vi "State Machine.vi"() -> ()   [LabVIEW 2015]
uses:
  Warning.ctl
  <vilib>/ErrorRing/Error Ring.xnode
panel:
  out "value voltage":dbl caption="Current Value (V)" format="%#.2g"
  out "Meter":dbl(knob) caption="Voltage" scale=0.0..12.0
  out "Low Link Quality Voltage":bool caption="Low"
  out "timed out?\nSignal potentiometer":bool caption="Timeout"
  out "Low Battery Voltage":bool caption="Low"
  out "timed out?\nBattery potentiometer":bool caption="Timeout"
  out "Signal > 75 %":bool
  out "Signal > 50 %":bool
  out "Signal > 25%":bool
  out "Signal > 0%":bool
  out "Battery > 75 %":bool
  out "Battery > 50 %":bool
  out "Battery > 25%":bool
  out "Battery > 0%":bool
  in  "upper and lower voltage threshold":cluster{dbl, dbl}(knob)={0.0, 12.0} caption="Voltage Threshold" scale=0.0..12.0
  out "Too High Voltage":bool
  out "Too Low Voltage":bool
  out "Low Link Quality Temp":bool caption="Low"
  out "timed out?\nLink Quality\nThermometer":bool caption="Timeout"
  out "Low Battery Temp":bool caption="Low"
  out "timed out?\nBattery Thermometer":bool caption="Timeout"
  out "Date":timestamp format="%<%d/%m/%y>T"
  out "Time":timestamp format="%<%H:%M>T"
  in  "Start/ pause":bool
  in  "Stop button":bool
  in  "upper and lower temp threshold":cluster{dbl, dbl}(knob)={0.0, 30.0} caption="Temperature Threshold" scale=-20.0..60.0
  out "Thermometer":dbl(slide) caption="Temperature" scale=-20.0..60.0
  in  "Error In":errorcluster
  out "Too hot":bool
  out "Too cold":bool
  out "min volt":sgl caption="Minimum (V)" format="%#.2g"
  out "max volt":sgl caption="Maximum (V)" format="%#.2g"
  out "mean volt":T1 caption="Mean (V)" format="%#.2g"
  out "voltage":sgl(graph)
  out "min temp":sgl caption="Minimum (°C)" format="%#.2g"
  out "max temp":sgl caption="Maximum (°C)" format="%#.2g"
  out "mean temp":sgl caption="Mean (°C)" format="%#.2g"
  out "temperature":sgl(graph)
  out "Signal > 75 % Temp":bool
  out "Signal > 50 % Temp":bool
  out "Signal > 25% Temp":bool
  out "Signal > 0% Temp":bool
  out "Battery > 75 % Temp":bool
  out "Battery > 50 % Temp":bool
  out "Battery > 25% Temp":bool
  out "Battery > 0% Temp":bool
  out "Low radio signal\nfor potentiometer":errorcluster
  out "Low Battery\nfor potentiometer":errorcluster
  out "No Signal \non thermometer":errorcluster
  out "No Signal\non potentiometer":errorcluster
  out "Low radio signal\nfor thermometer":errorcluster
  out "Low Battery\nfor thermometer":errorcluster
  # "Thermometer"
  # "Potentiometer"
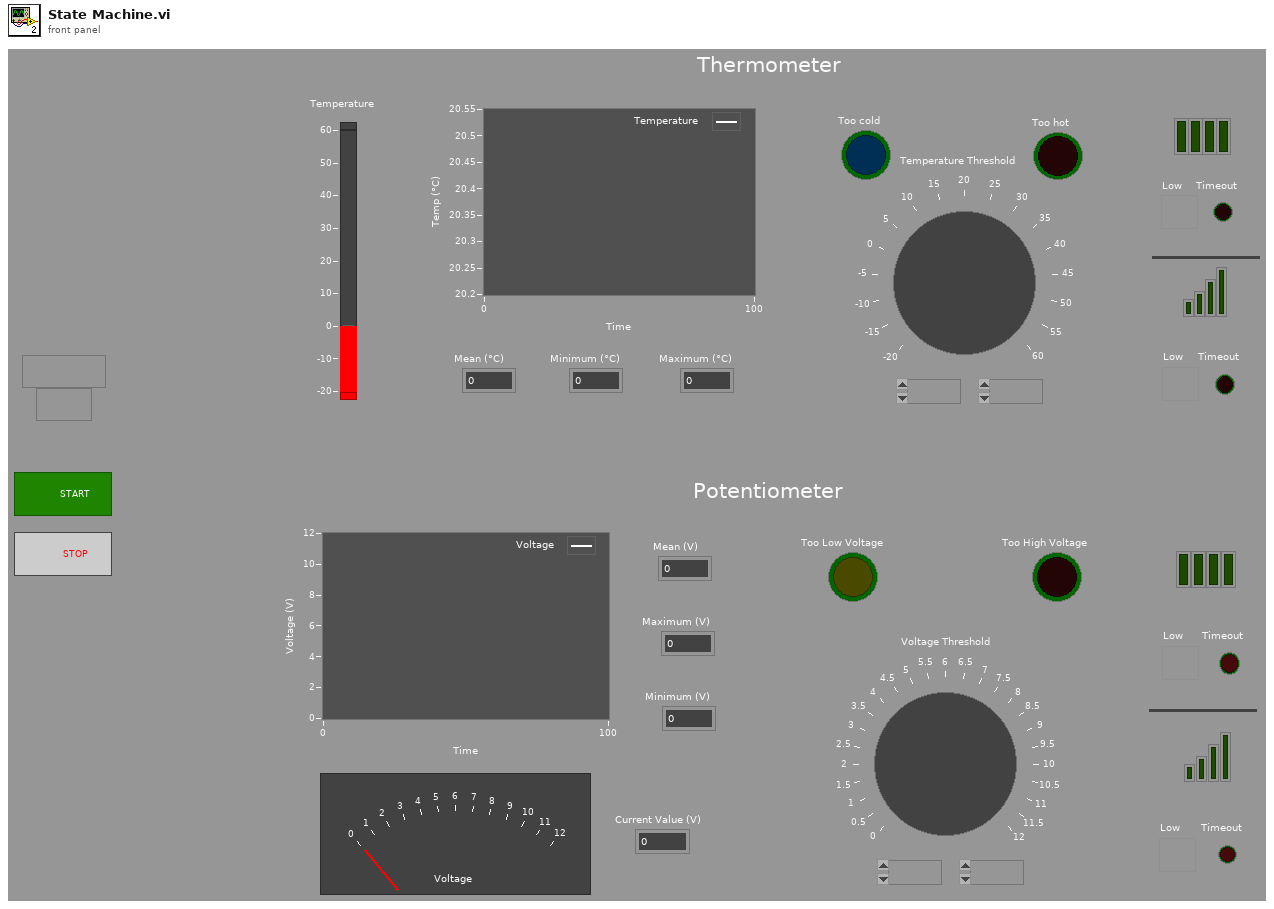
[diagram p1: front panel]
types:
  T1 = typedef "Warning.ctl" = sgl
  T2 = enum16{"open", "replace", "create", "open or create", "replace or create", "replace or create with confirmation"}
  T3 = enum8{"Enabled", "Disabled", "Disabled and Grayed Out"}
  T4 = enum16{"Error and Alert handler", "Acquisition, calculations and save"}
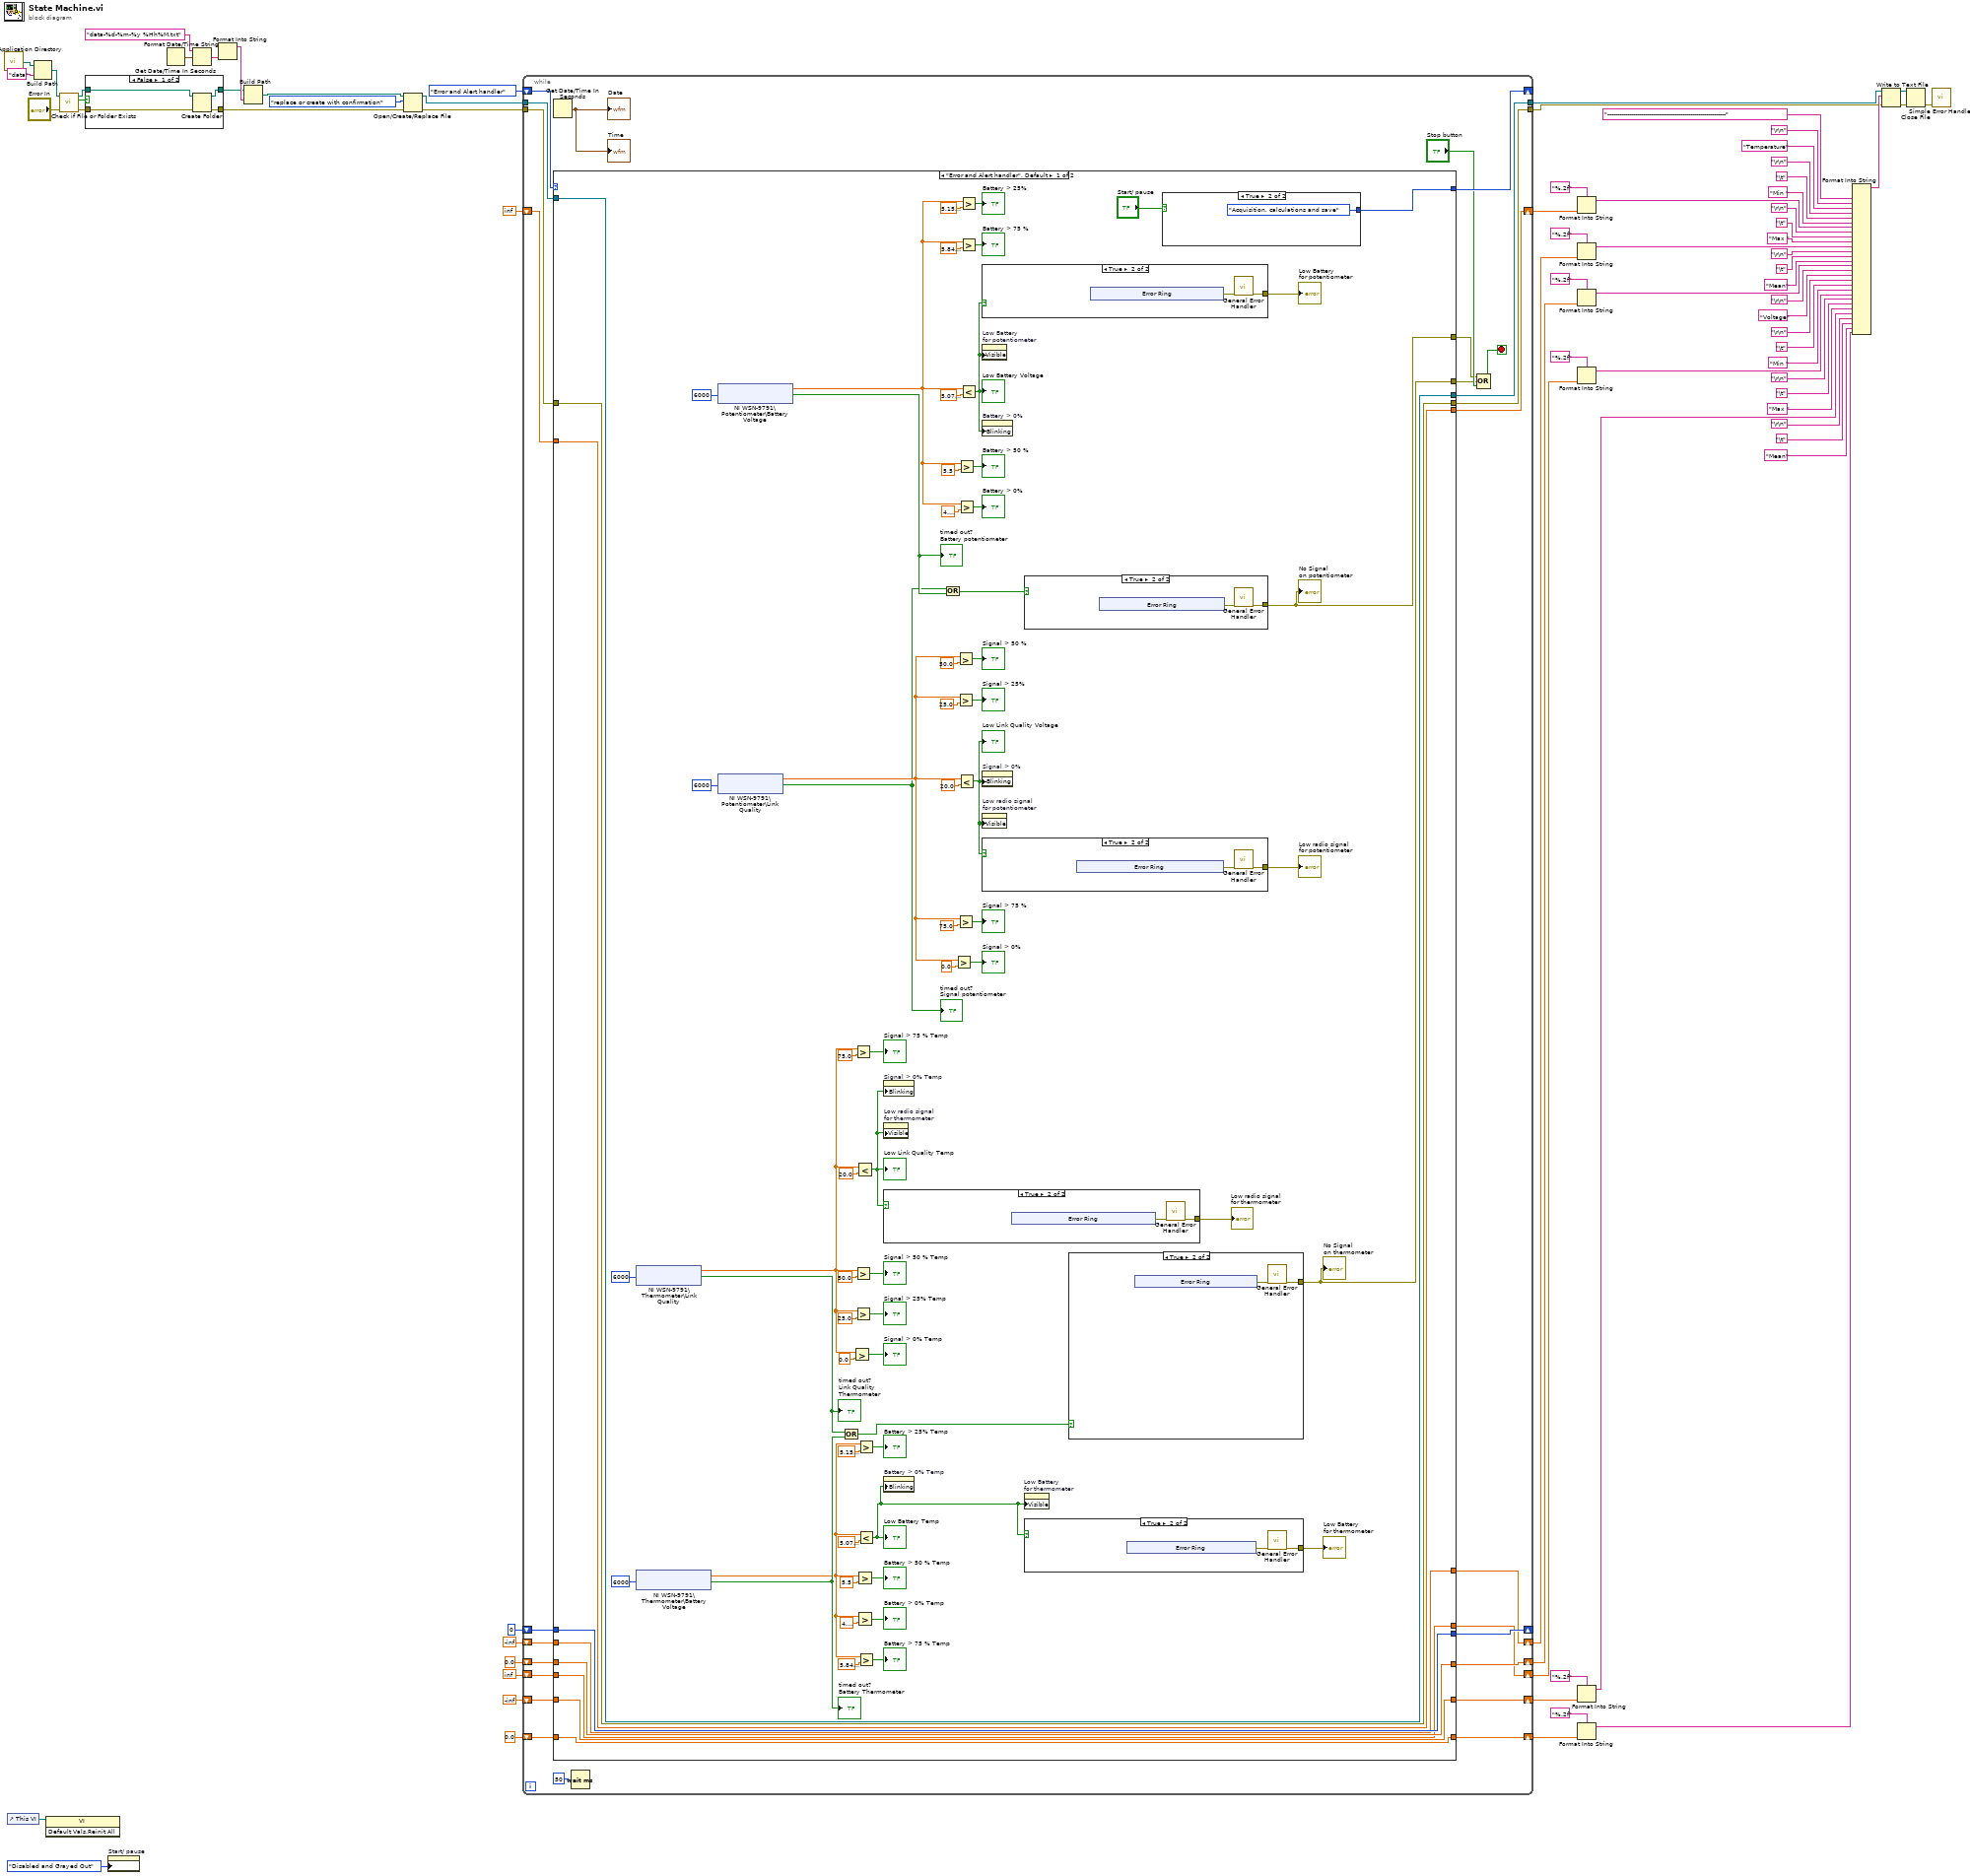
[diagram p0: block diagram]
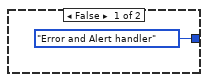
[diagram p3: hidden frame]
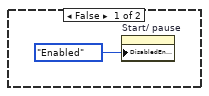
[diagram p7: hidden frame]
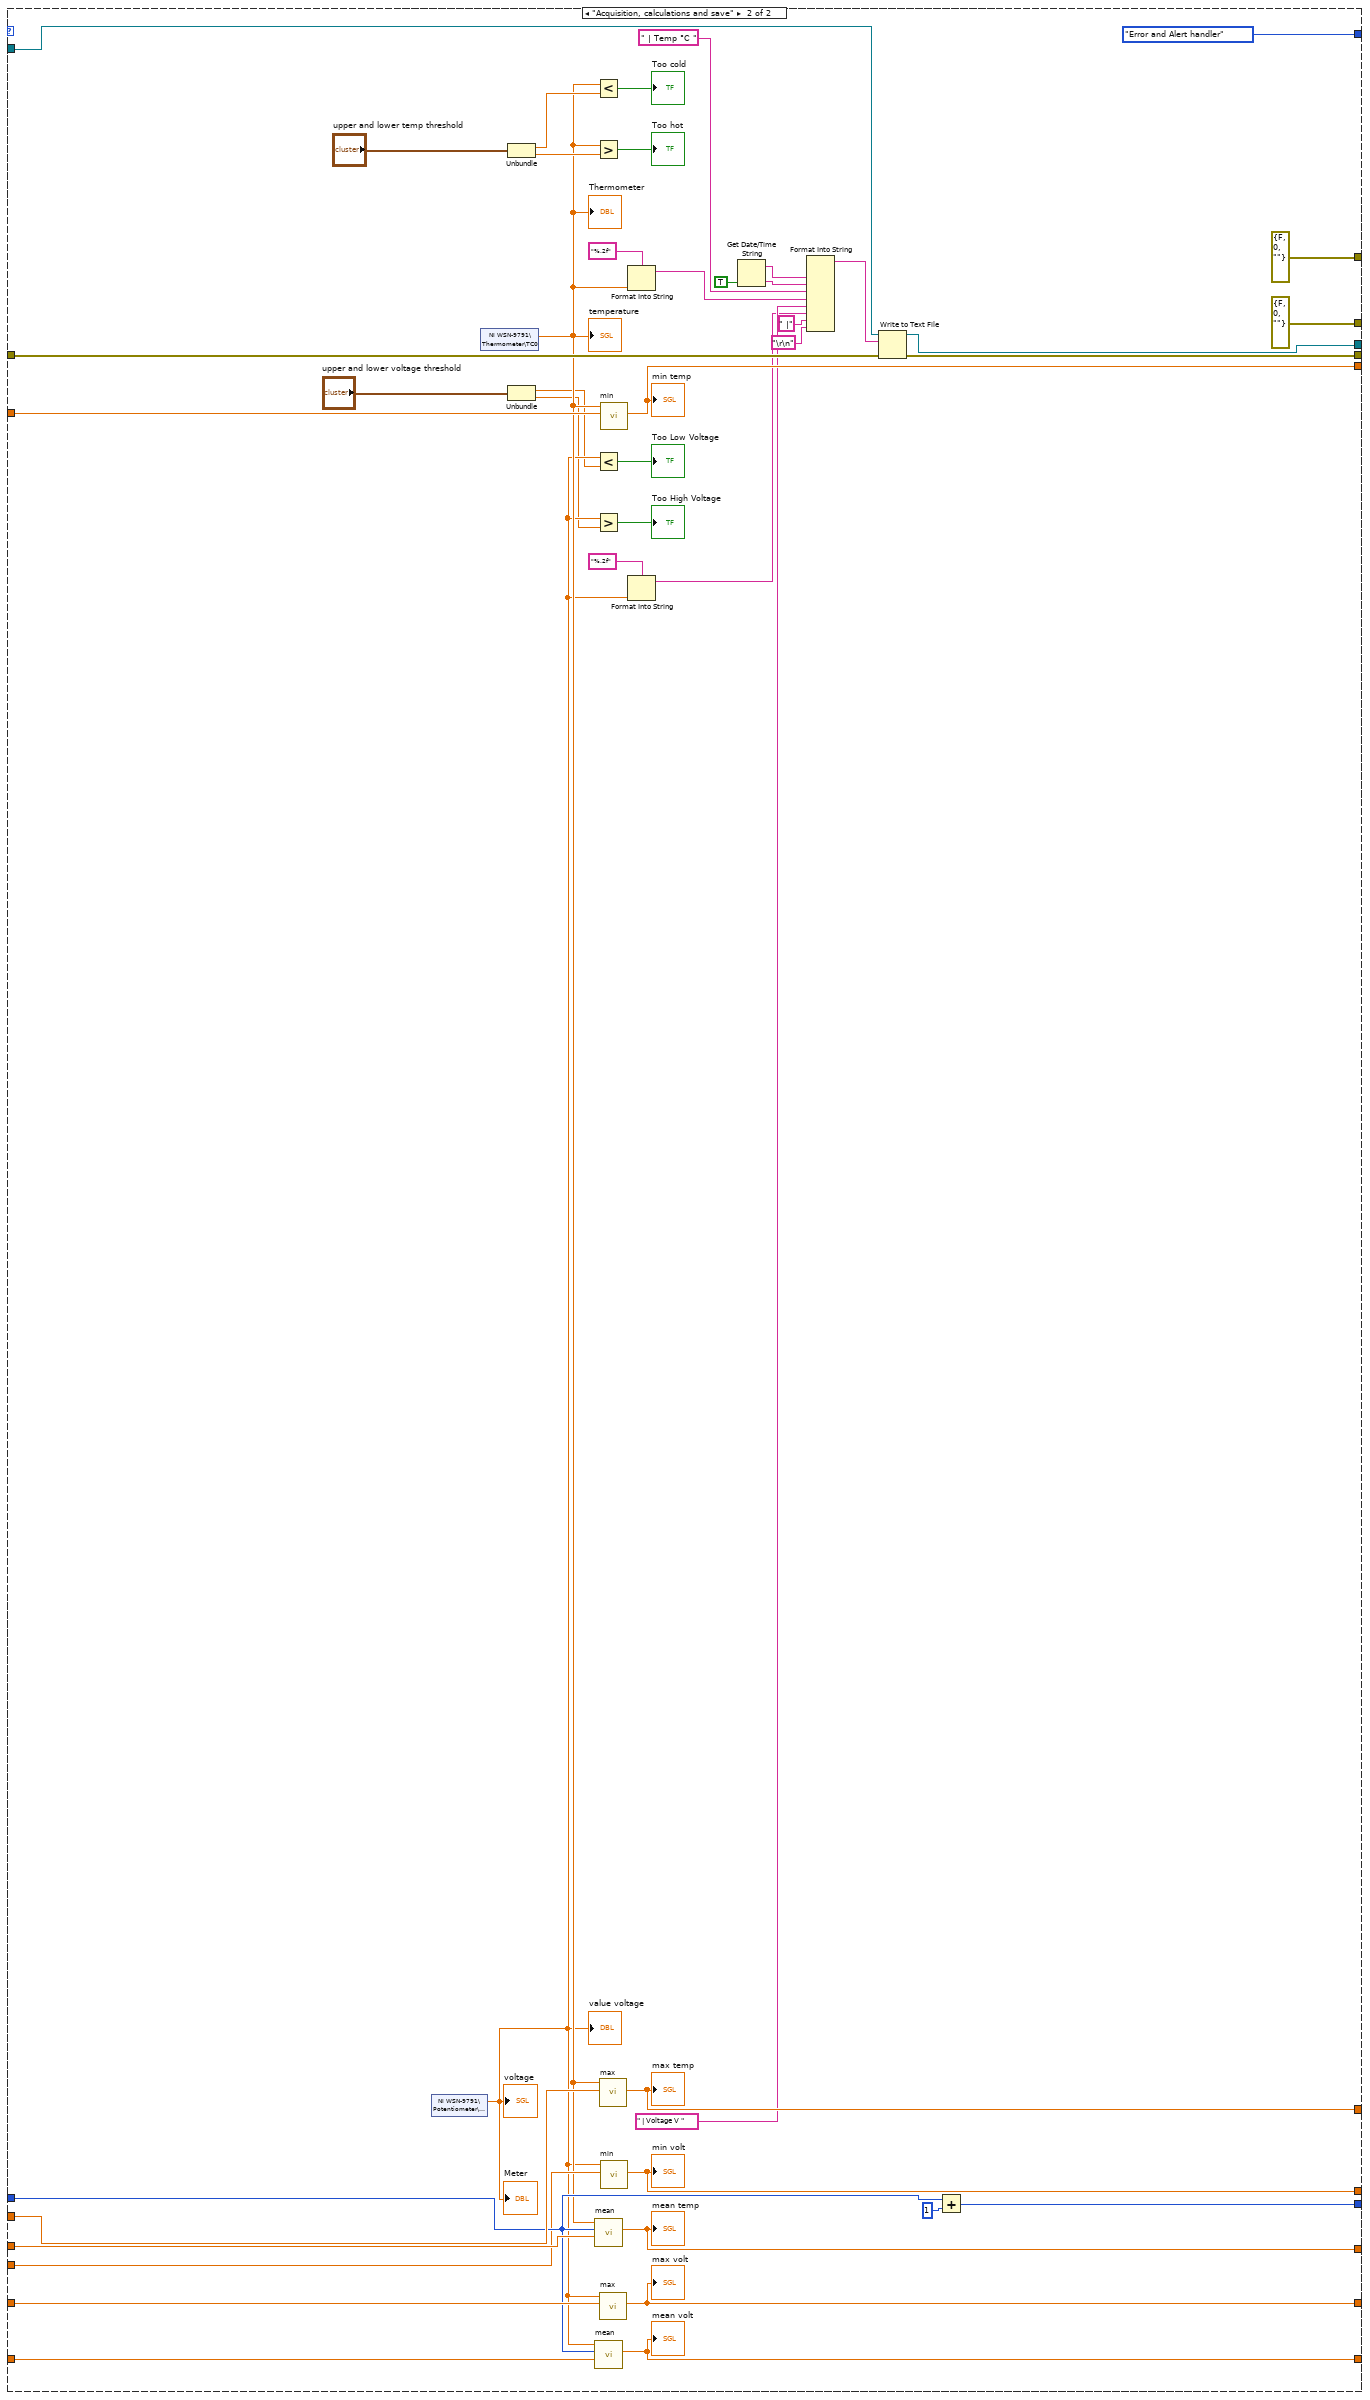
[diagram p10: hidden frame]
diagram:
  n1 = call <vilib>:"Application Directory.vi"() -> ("Application Directory"=w12:path)
  n2 = control-ref of="This VI"() -> (w1:refnum<vi>)
  n3 = Build Path(base path=w12, name or relative path="data") -> (appended path=w8:path)
  n4 = invoke class="VI" method="Default Vals.Reinit All"(reference=w1) -> ()  [unwired: 2 in, 3 out]
  n5 = call <vilib>:"Check if File or Folder Exists.vi"("error in (no error)"="Error In", "path"=w8) -> ("error out"=w6:errorcluster, "file or folder exists?"=w7:bool, "dup path"=w4:path)  [unwired: 7 in]
  n6 = case shown="False" w7 {
    tunnel: w6 -> [w78 w79]
    tunnel: [w77 w79] -> w5
    tunnel: w4 -> [w76 w80]
    tunnel: [w75 w80] -> w3
    frame False {
      n7 = Create Folder(path (use dialog)=w76, error in=w78) -> (created path=w75:path, error out=w77:errorcluster)  [unwired: 1 in, 1 out]
    }
    frame True {
    }
  }
  n8 = property on="Start/ pause" class="Bool (strict)"("DisabledEnum"=T3."Disabled and Grayed Out" ("Disabled")) -> ()  [unwired: 2 in, 2 out]
  n9 = Get Date/Time In Seconds() -> (seconds since 1Jan1904=w15:timestamp)
  n10 = Format Date/Time String(time format string (%c)="data-%d-%m-%y %Hh%M.txt", seconds (now)=w15) -> (date/time string=w13:string)  [unwired: 1 in]
  n11 = Format Into String(w13) -> (resulting string=w10:string)  [unwired: 3 in, 1 out]
  n12 = Build Path(base path=w3, name or relative path=w10) -> (appended path=w9:path)
  n13 = Open/Create/Replace File(file path (use dialog)=w9, error in=w5, operation (0:open)=T2."replace or create with confirmation") -> (refnum out=w60:refnum<file>, error out=w57:errorcluster)  [unwired: 3 in, 1 out]
  n14 = while {
    shift-right: [w105] -> _
    shift-left: T4."Error and Alert handler" -> [w101]
    shift-right: [w99] -> _
    shift-left: 0 -> [w100]
    shift-right: [w97] -> w37
    shift-left: sgl 0.0 -> [w98]
    shift-right: [w95] -> w36
    shift-left: -inf -> [w96]
    shift-right: [w93] -> w44
    shift-left: inf -> [w94]
    shift-right: [w89] -> w16
    shift-left: sgl 0.0 -> [w90]
    shift-right: [w88] -> w17
    shift-left: -inf -> [w91]
    shift-right: [w87] -> w18
    shift-left: inf -> [w92]
    tunnel: w60 -> [w85]
    tunnel: [w84] -> w59
    tunnel: [w83] -> w58
    tunnel: w57 -> [w82]
    stop <- w86 stop-if-true
    n15 = Get Date/Time In Seconds() -> (seconds since 1Jan1904=→"Time" →"Date":timestamp)
    n16 = case shown="\"Error and Alert handler\", Default" w101 {
      tunnel: [w118 T4."Error and Alert handler"] -> w105
      tunnel: [w132 errorcluster {"status"=FALSE, "code"=0, "source"=""} ("error out")] -> w103
      tunnel: [w131 errorcluster {"status"=FALSE, "code"=0, "source"=""} ("error out")] -> w102
      tunnel: w100 -> [w126 w231]
      tunnel: [w126 w229] -> w99
      tunnel: w98 -> [w125 w241]
      tunnel: [w125 w240] -> w97
      tunnel: w96 -> [w124 w239]
      tunnel: [w124 w237] -> w95
      tunnel: w94 -> [w123 w238]
      tunnel: [w123 w236] -> w93
      tunnel: w92 -> [w120 w228]
      tunnel: w91 -> [w121 w235]
      tunnel: w90 -> [w122 w234]
      tunnel: [w122 w233] -> w89
      tunnel: [w121 w232] -> w88
      tunnel: [w120 w227] -> w87
      tunnel: w85 -> [w117 w222]
      tunnel: [w117 w221] -> w84
      tunnel: [w116 w220] -> w83
      tunnel: w82 -> [w116 w219]
      frame "Error and Alert handler", Default {
        n17 = shared-variable "NI WSN-9791\\Thermometer\\Link Quality"(6000 ("ms timeout (0)")) -> (w112:sgl, w129:bool)  [unwired: 1 in, 1 out]
        "timed out?\nLink Quality\nThermometer" <- w129
        n18 = shared-variable "NI WSN-9791\\Thermometer\\Battery Voltage"(6000 ("ms timeout (0)")) -> (w113:sgl, w130:bool)  [unwired: 1 in, 1 out]
        "timed out?\nBattery Thermometer" <- w130
        n19 = shared-variable "NI WSN-9791\\Potentiometer\\Battery Voltage"(6000 ("ms timeout (0)")) -> (w111:sgl, w128:bool)  [unwired: 1 in, 1 out]
        "timed out?\nBattery potentiometer" <- w128
        n20 = shared-variable "NI WSN-9791\\Potentiometer\\Link Quality"(6000 ("ms timeout (0)")) -> (w133:sgl, w127:bool)  [unwired: 1 in, 1 out]
        "timed out?\nSignal potentiometer" <- w127
        n21 = Or(x=w129, y=w130) -> (x .or. y?=w174:bool)
        n22 = Greater?(x=w112, y=sgl 0.0) -> (0:→"Signal > 0% Temp":bool)
        n23 = Greater?(x=w112, y=sgl 75.0) -> (0:→"Signal > 75 % Temp":bool)
        n24 = Greater?(x=w112, y=sgl 50.0) -> (0:→"Signal > 50 % Temp":bool)
        n25 = Greater?(x=w112, y=sgl 25.0) -> (0:→"Signal > 25% Temp":bool)
        n26 = Less?(x=w112, y=sgl 20.0) -> (x < y?=w108:bool)
        "Low Link Quality Temp" <- w108
        n27 = Greater?(x=w113, y=sgl 5.5) -> (0:→"Battery > 50 % Temp":bool)
        n28 = Greater?(x=w113, y=sgl 4.8) -> (0:→"Battery > 0% Temp":bool)
        n29 = Greater?(x=w113, y=sgl 5.15) -> (0:→"Battery > 25% Temp":bool)
        n30 = Less?(x=w113, y=sgl 5.08) -> (x < y?=w107:bool)
        "Low Battery Temp" <- w107
        n31 = Greater?(x=w113, y=sgl 5.85) -> (0:→"Battery > 75 % Temp":bool)
        n32 = property on="Signal > 0% Temp" class="Bool (strict)"("Blinking"=w108) -> ()  [unwired: 2 in, 2 out]
        n33 = property on="Low radio signal\nfor thermometer" class="Clust (strict)"("Visible"=w108) -> ()  [unwired: 2 in, 2 out]
        n34 = case shown="True" w108 {
          tunnel: [_ w194] -> w176
          frame False {
          }
          frame True {
            n35 = xnode "Error Ring"() -> ("error out"=w193:errorcluster)
            n36 = call <vilib>:"General Error Handler.vi"("error in (no error)"=w193) -> ("error out"=w194:errorcluster)  [unwired: 10 in, 4 out]
          }
        }
        "Low radio signal\nfor thermometer" <- w176
        n37 = property on="Battery > 0% Temp" class="Bool (strict)"("Blinking"=w107) -> ()  [unwired: 2 in, 2 out]
        n38 = Or(x=w127, y=w128) -> (x .or. y?=w175:bool)
        n39 = Greater?(x=w133, y=sgl 0.0) -> (0:→"Signal > 0%":bool)
        n40 = Greater?(x=w133, y=sgl 50.0) -> (0:→"Signal > 50 %":bool)
        n41 = Greater?(x=w133, y=sgl 25.0) -> (0:→"Signal > 25%":bool)
        n42 = Greater?(x=w133, y=sgl 75.0) -> (0:→"Signal > 75 %":bool)
        n43 = Greater?(x=w111, y=sgl 5.5) -> (0:→"Battery > 50 %":bool)
        n44 = Greater?(x=w111, y=sgl 4.8) -> (0:→"Battery > 0%":bool)
        n45 = Less?(x=w133, y=sgl 20.0) -> (x < y?=w110:bool)
        "Low Link Quality Voltage" <- w110
        n46 = Greater?(x=w111, y=sgl 5.15) -> (0:→"Battery > 25%":bool)
        n47 = Greater?(x=w111, y=sgl 5.85) -> (0:→"Battery > 75 %":bool)
        n48 = Less?(x=w111, y=sgl 5.08) -> (x < y?=w109:bool)
        "Low Battery Voltage" <- w109
        n49 = case shown="True" w109 {
          tunnel: [_ w184] -> w173
          frame False {
          }
          frame True {
            n50 = xnode "Error Ring"() -> ("error out"=w183:errorcluster)
            n51 = call <vilib>:"General Error Handler.vi"("error in (no error)"=w183) -> ("error out"=w184:errorcluster)  [unwired: 10 in, 4 out]
          }
        }
        "Low Battery\nfor potentiometer" <- w173
        n52 = property on="Low Battery\nfor potentiometer" class="Clust (strict)"("Visible"=w109) -> ()  [unwired: 2 in, 2 out]
        n53 = property on="Battery > 0%" class="Bool (strict)"("Blinking"=w109) -> ()  [unwired: 2 in, 2 out]
        n54 = property on="Signal > 0%" class="Bool (strict)"("Blinking"=w110) -> ()  [unwired: 2 in, 2 out]
        n55 = property on="Low radio signal\nfor potentiometer" class="Clust (strict)"("Visible"=w110) -> ()  [unwired: 2 in, 2 out]
        n56 = case shown="True" w110 {
          tunnel: [_ w181] -> w172
          frame False {
          }
          frame True {
            n57 = xnode "Error Ring"() -> ("error out"=w180:errorcluster)
            n58 = call <vilib>:"General Error Handler.vi"("error in (no error)"=w180) -> ("error out"=w181:errorcluster)  [unwired: 10 in, 4 out]
          }
        }
        "Low radio signal\nfor potentiometer" <- w172
        n59 = case shown="True" w175 {
          tunnel: [_ w191] -> w131
          frame False {
            n60 = property on="Start/ pause" class="Bool (strict)"("DisabledEnum"=T3."Enabled" ("Disabled")) -> ()  [unwired: 2 in, 2 out]
          }
          frame True {
            n61 = xnode "Error Ring"() -> ("error out"=w190:errorcluster)
            n62 = call <vilib>:"General Error Handler.vi"("error in (no error)"=w190) -> ("error out"=w191:errorcluster)  [unwired: 10 in, 4 out]
          }
        }
        "No Signal\non potentiometer" <- w131
        n63 = property on="Low Battery\nfor thermometer" class="Clust (strict)"("Visible"=w107) -> ()  [unwired: 2 in, 2 out]
        n64 = case shown="True" w107 {
          tunnel: [_ w197] -> w177
          frame False {
          }
          frame True {
            n65 = xnode "Error Ring"() -> ("error out"=w196:errorcluster)
            n66 = call <vilib>:"General Error Handler.vi"("error in (no error)"=w196) -> ("error out"=w197:errorcluster)  [unwired: 10 in, 4 out]
          }
        }
        "Low Battery\nfor thermometer" <- w177
        n67 = case shown="True" w174 {
          tunnel: [_ w187] -> w132
          frame False {
          }
          frame True {
            n68 = xnode "Error Ring"() -> ("error out"=w186:errorcluster)
            n69 = call <vilib>:"General Error Handler.vi"("error in (no error)"=w186) -> ("error out"=w187:errorcluster)  [unwired: 10 in, 4 out]
          }
        }
        "No Signal \non thermometer" <- w132
        n70 = case shown="True" "Start/ pause" {
          tunnel: [T4."Error and Alert handler" T4."Acquisition, calculations and save"] -> w118
          frame False {
          }
          frame True {
          }
        }
      }
      frame "Acquisition, calculations and save" {
        n71 = shared-variable "NI WSN-9791\\Potentiometer\\AI0"() -> (w201:sgl)  [unwired: 1 in, 1 out]
        "voltage" <- w201
        "value voltage" <- w201
        "Meter" <- w201
        n72 = shared-variable "NI WSN-9791\\Thermometer\\TC0"() -> (w202:sgl)  [unwired: 1 in, 1 out]
        "temperature" <- w202
        "Thermometer" <- w202
        n73 = Unbundle("upper and lower temp threshold") -> (w203:dbl, w204:dbl)
        n74 = Unbundle("upper and lower voltage threshold") -> (w199:dbl, w200:dbl)
        n75 = Less?(x=w202, y=w203) -> (x < y?=→"Too cold":bool)
        n76 = Greater?(x=w202, y=w204) -> (0:→"Too hot":bool)
        n77 = Less?(x=w201, y=w199) -> (x < y?=→"Too Low Voltage":bool)
        n78 = Greater?(x=w201, y=w200) -> (0:→"Too High Voltage":bool)
        n79 = call "mean.vi"("Numeric 2"=w241, "n"=w231, "Numeric"=w202) -> ("mean"=w240:sgl)  [unwired: 8 in]
        "mean temp" <- w240
        n80 = call "mean.vi"("Numeric 2"=w234, "n"=w231, "Numeric"=w201) -> ("mean"=w233:sgl)  [unwired: 8 in]
        "mean volt" <- w233
        n81 = call "max.vi"("Numeric 3"=w239, "Numeric in"=w202) -> ("max"=w237:sgl)  [unwired: 9 in]
        "max temp" <- w237
        n82 = call "max.vi"("Numeric 3"=w235, "Numeric in"=w201) -> ("max"=w232:sgl)  [unwired: 9 in]
        "max volt" <- w232
        n83 = call "min.vi"("Numeric"=w238, "Numeric 2"=w202) -> ("min"=w236:sgl)  [unwired: 9 in]
        "min temp" <- w236
        n84 = call "min.vi"("Numeric"=w228, "Numeric 2"=w201) -> ("min"=w227:sgl)  [unwired: 9 in]
        "min volt" <- w227
        n85 = Format Into String(format string="%.2f", w202) -> (resulting string=w207:string)  [unwired: 2 in, 1 out]
        n86 = Format Into String(format string="%.2f", w201) -> (resulting string=w209:string)  [unwired: 2 in, 1 out]
        n87 = Get Date/Time String(want seconds? (F)=TRUE) -> (date string=w217:string, time string=w216:string)  [unwired: 2 in]
        n88 = Format Into String(w217, w216, " | Temp °C " ("input 3"), w207, " | Voltage V " ("input 5"), w209, " |" ("input 7"), "\r\n") -> (resulting string=w218:string)  [unwired: 3 in, 1 out]
        n89 = Write to Text File(file (use dialog)=w222, text=w218, error in=w219) -> (refnum out=w221:refnum<file>, error out=w220:errorcluster)  [unwired: 1 in, 1 out]
        n90 = Add(x=w231, y=1) -> (x+y=w229:i32)
      }
    }
    n91 = Wait (ms)(milliseconds to wait=u32 50) -> ()  [unwired: 1 out]
    n92 = Compound Arithmetic op=OR(w102, w103, "Stop button") -> (w86:bool)
  }
  n93 = Format Into String(format string="%.2f", w44) -> (resulting string=w42:string)  [unwired: 2 in, 1 out]
  n94 = Format Into String(format string="%.2f", w36) -> (resulting string=w40:string)  [unwired: 2 in, 1 out]
  n95 = Format Into String(format string="%.2f", w37) -> (resulting string=w38:string)  [unwired: 2 in, 1 out]
  n96 = Format Into String(format string="%.2f", w18) -> (resulting string=w29:string)  [unwired: 2 in, 1 out]
  n97 = Format Into String(format string="%.2f", w17) -> (resulting string=w24:string)  [unwired: 2 in, 1 out]
  n98 = Format Into String(format string="%.2f", w16) -> (resulting string=w19:string)  [unwired: 2 in, 1 out]
  n99 = Format Into String("------------------------------------------------------------" ("input 1"), "\r\n", "Temperature" ("input 1"), "\r\n", "\t", "Min " ("input 1"), w42, "\r\n", "\t", "Max " ("input 1"), w40, "\r\n", "\t", "Mean" ("input 1"), w38, "\r\n", "Voltage" ("input 1"), "\r\n", "\t", "Min " ("input 1"), w29, "\r\n", "\t", "Max " ("input 1"), w24, "\r\n", "\t", "Mean" ("input 1"), w19) -> (resulting string=w61:string)  [unwired: 3 in, 1 out]
  n100 = Write to Text File(file (use dialog)=w59, text=w61, error in=w58) -> (refnum out=w63:refnum<file>, error out=w62:errorcluster)  [unwired: 1 in, 1 out]
  n101 = Close File(refnum=w63, error in=w62) -> (error out=w64:errorcluster)  [unwired: 1 out]
  n102 = call <vilib>:"Simple Error Handler.vi"("error in (no error)"=w64) -> ()  [unwired: 4 in, 5 out]
